vi "ReadMultiMeter.vi"(2 "Measeaurement mode":string(combo), 3 "Input Device":refnum<visa-resource-name>) -> (0 "Volt":dbl=-0.056988192, 1 "VISA Resource Name out":refnum<visa-resource-name>="GPIB0::22::INSTR")   [LabVIEW 2011]
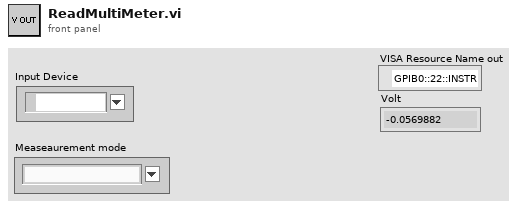
[diagram p1: front panel]
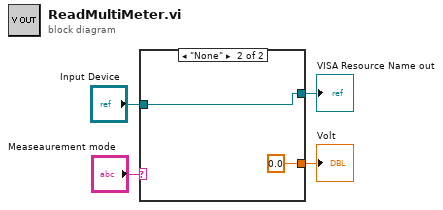
[diagram p0: block diagram]
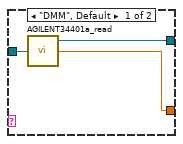
[diagram p2: hidden frame]
diagram:
  n1 = case shown="\"None\"" "Measeaurement mode" {
    tunnel: "Input Device" -> [w7 w8]
    tunnel: [w6 w8] -> w2
    tunnel: [w5 0.0 ("Voltage output")] -> w1
    frame "DMM", Default {
      n2 = call "AGILENT34401a_read.vi"("VISA Resource Name in"=w7) -> ("VISA Resource Name out"=w6:refnum<visa-resource-name>, "Voltage output"=w5:dbl)  [unwired: 1 out]
    }
    frame "None" {
    }
  }
  "VISA Resource Name out" <- w2
  "Volt" <- w1
